vi "control panel decoration exercise.vi"() -> ()   [LabVIEW 2024]
panel:
  out "Random input x":dbl
  out "Answer y":dbl
  out "No of loop":i32
  in  "stop":bool
  out "Is square bigger than circle?":bool
  out "Square Area":dbl
  in  "Side":dbl
  out "Area":dbl
  in  "r":dbl
  in  "Boolean 8":bool
  in  "Boolean 7":bool
  in  "Boolean 6":bool
  in  "Boolean 5":bool
  out "Boolean 4":bool
  out "Boolean 3":bool
  out "Boolean 2":bool
  out "Boolean":bool
  out "Numeric  indicator 4":dbl
  out "Numeric  indicator 3":dbl
  out "Numeric  indicator 2":dbl
  out "Numeric  indicator":dbl
  in  "Numeric 4":u16
  in  "Numeric 3":i32
  in  "Numeric 2":dbl
  in  "Numeric":u8
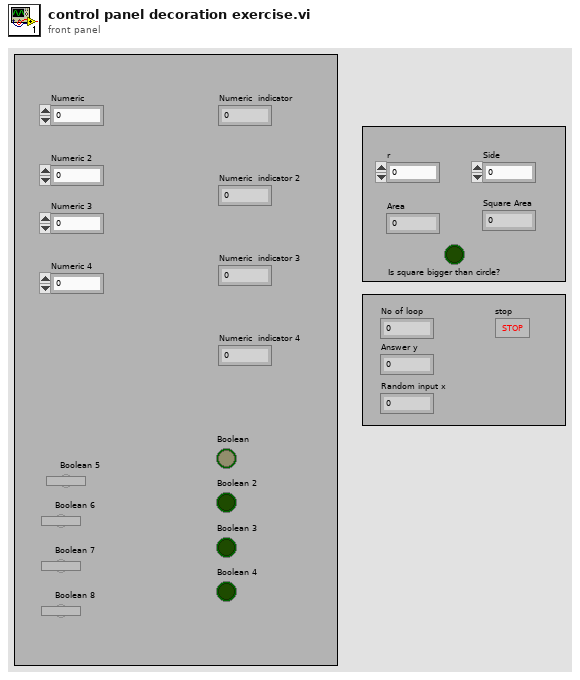
[diagram p1: front panel]
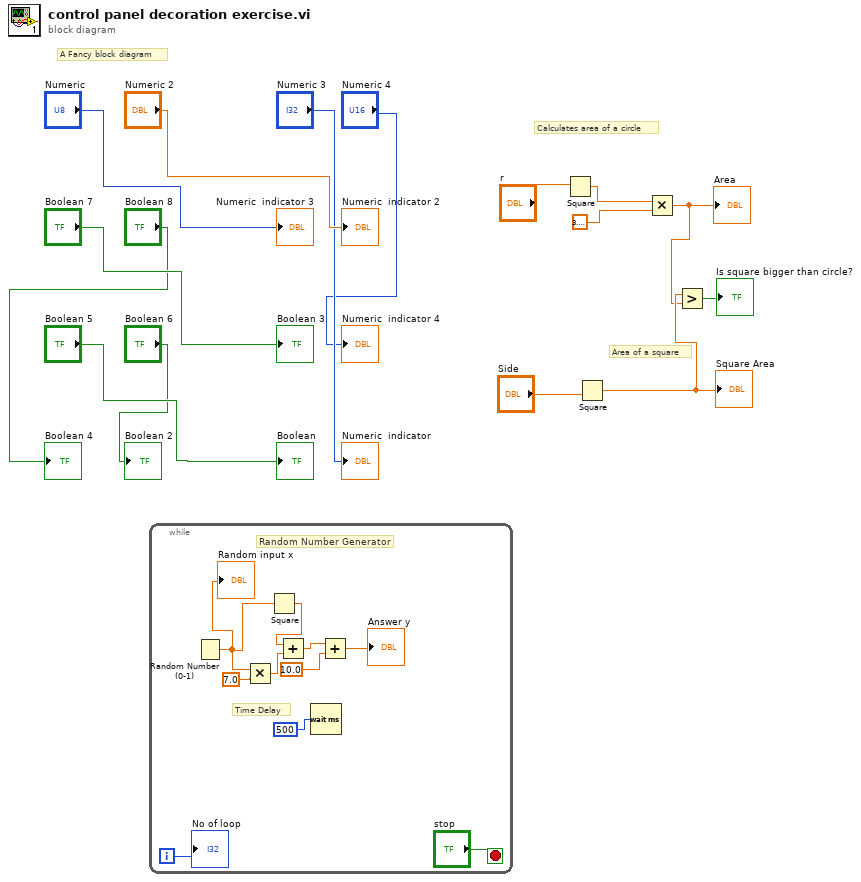
[diagram p0: block diagram]
diagram:
  # "Area of a square"
  # "Calculates area of a circle"
  # "A Fancy block diagram"
  n1 = while {
    i -> [w24]
    stop <- "stop" stop-if-true
    # "Time Delay"
    # "Random Number Generator"
    n2 = Random Number (0-1)() -> (number: 0 to 1=w16:dbl)
    "Random input x" <- w16
    n3 = Multiply(x=w16, y=7.0) -> (x*y=w22:dbl)
    n4 = Square(x=w16) -> (x^2=w20:dbl)
    n5 = Add(x=w20, y=w22) -> (x+y=w19:dbl)
    n6 = Wait (ms)(milliseconds to wait=u32 500 ("millisecond timer value")) -> ()  [unwired: 1 out]
    n7 = Add(x=w19, y=10.0) -> (x+y=→"Answer y":dbl)
    "No of loop" <- w24
  }
  n8 = Square(x="r") -> (x^2=w6:dbl)
  n9 = Square(x="Side") -> (x^2=w2:dbl)
  "Square Area" <- w2
  n10 = Multiply(x=w6, y=3.141592653589793) -> (x*y=w1:dbl)
  "Area" <- w1
  n11 = Greater?(x=w2, y=w1) -> (0:→"Is square bigger than circle?":bool)
  "Numeric  indicator" <- "Numeric 3"
  "Numeric  indicator 2" <- "Numeric 2"
  "Numeric  indicator 3" <- "Numeric"
  "Numeric  indicator 4" <- "Numeric 4"
  "Boolean" <- "Boolean 5"
  "Boolean 2" <- "Boolean 6"
  "Boolean 3" <- "Boolean 7"
  "Boolean 4" <- "Boolean 8"
